vi "main.vi"() -> ()   [LabVIEW 2021]
uses:
  <extravilib>/ChannelInstances/Stream-c(dbl,dbl)/Read With Abort.vi
  <extravilib>/ChannelInstances/Stream-c(dbl,dbl)/Write With Abort.vi
  <extravilib>/ChannelInstances/Stream-c(dbl,dbl)/EndpointRead.vi
  <extravilib>/ChannelInstances/Stream-c(dbl,dbl)/Endpoint.vi
  <vilib>/Instr/_visa.llb/VISA Configure Serial Port (Instr).vi
  <extravilib>/ChannelInstances/Event Messenger-c(str)/Instantiate.vi
  <extravilib>/ChannelInstances/Event Messenger-c(str)/))Channel.vi
  <extravilib>/ChannelInstances/Stream-c(dbl,dbl)/Instantiate.vi
  <extravilib>/ChannelInstances/Stream-c(dbl,dbl)/)Channel.vi
  <resource>/ChannelSupport/_ChannelSupport/WaitIfNeeded.vi
  <extravilib>/ChannelInstances/Stream-c(dbl,dbl).lvlib
  <extravilib>/ChannelInstances/Event Messenger-c(str).lvlib
panel:
  in  "Start":bool
  out "File Path":path
  out "Recording?":bool
  in  "Record?":bool
  out "XY Graph":cluster{"X":dbl, "Y":dbl}[](graph)
  out "Temp":dbl
  out "Time":dbl
  in  "VISA resource name":refnum<visa-resource-name>
  in  "Stop":bool
  # "Select the VISA resource name before starting the application, you can choose to record to a file at any time using the checkbox. Data acquisition begins after you press Start."
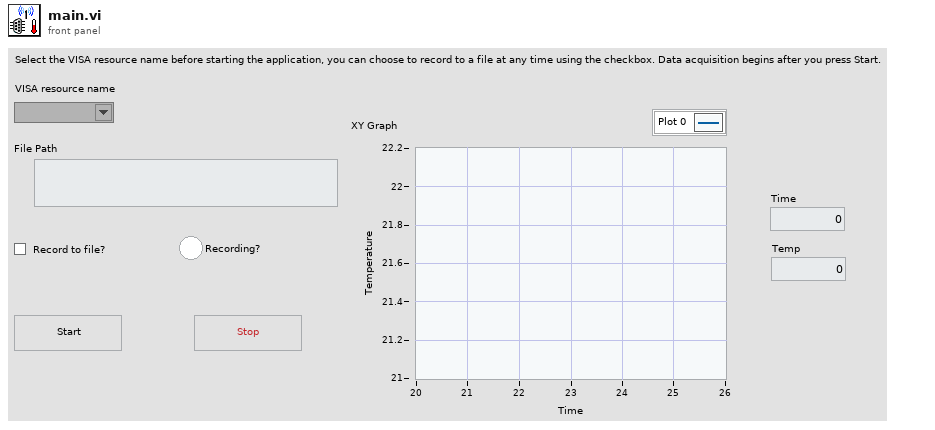
[diagram p1: front panel]
types:
  T1 = enum16{"open", "replace", "create", "open or create", "replace or create", "replace or create with confirmation"}
  T2 = typedef "Event Messenger-c(str).lvlib/))Channel.ctl" = refnum<queue>
  T3 = typedef "Stream-c(dbl,dbl).lvlib/)Channel.ctl" = refnum<queue>
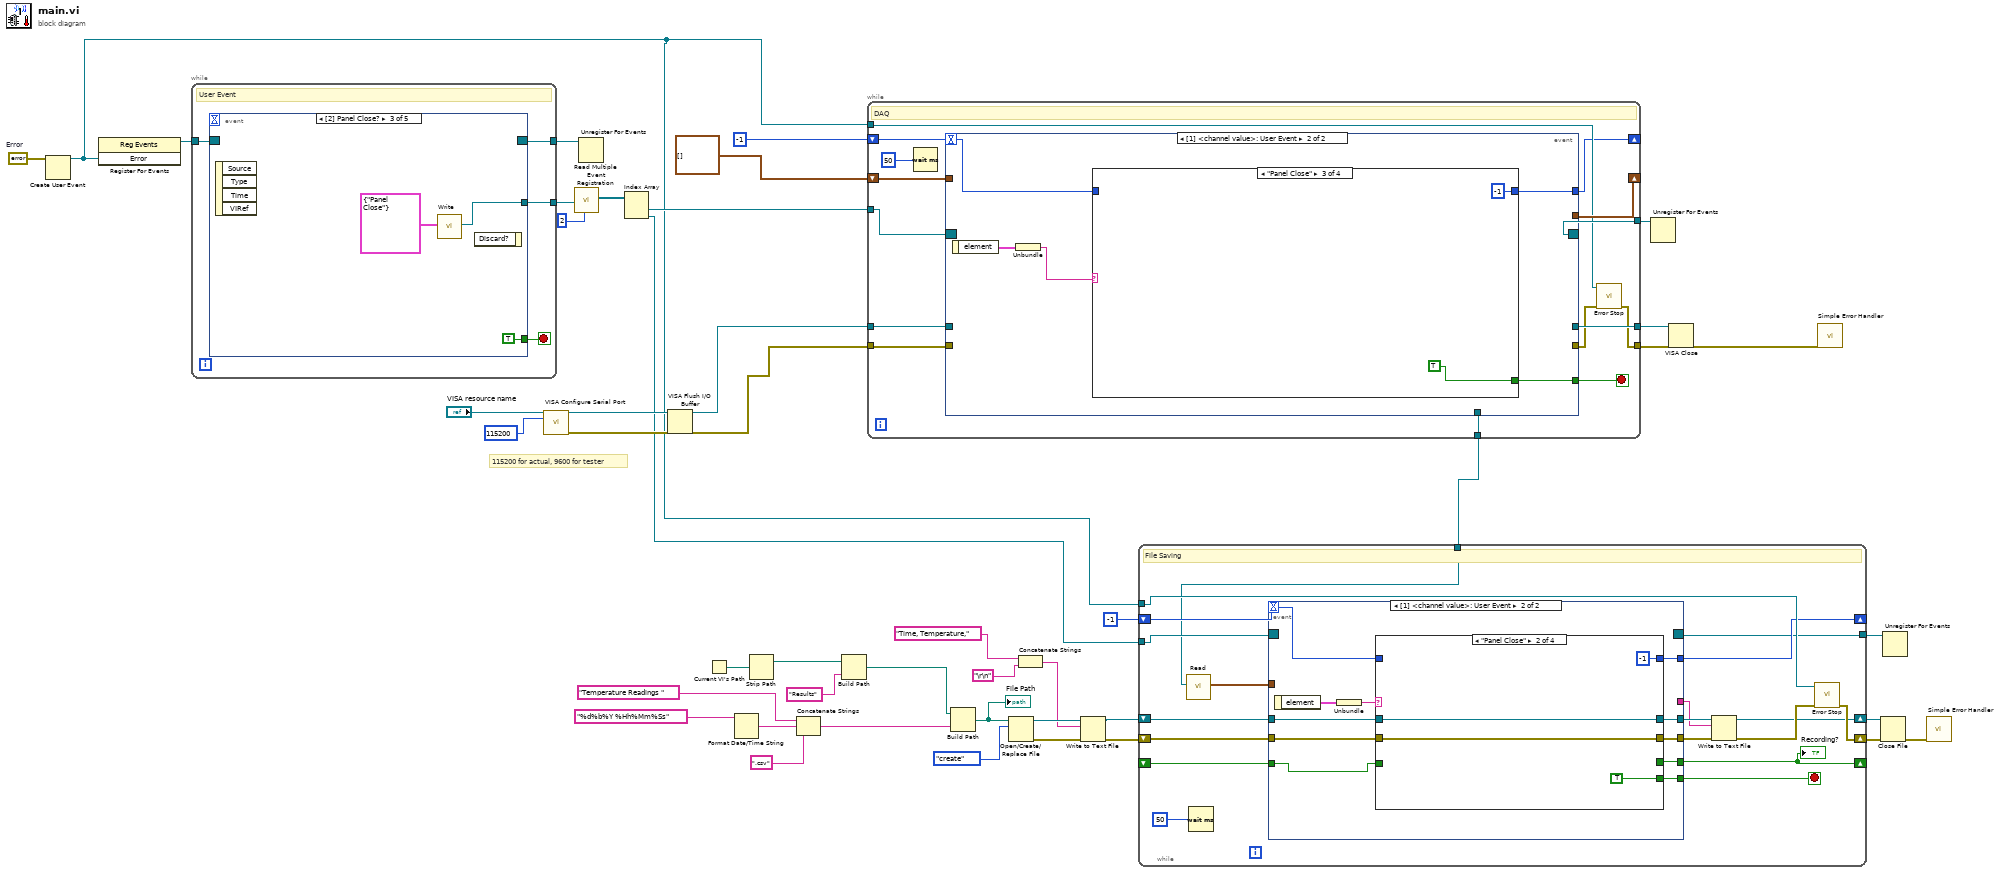
[diagram p0: block diagram]
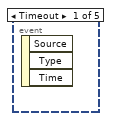
[diagram p2: hidden frame]
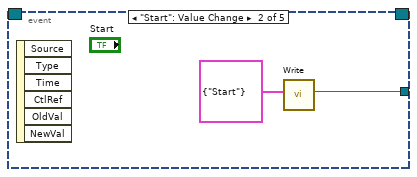
[diagram p3: hidden frame]
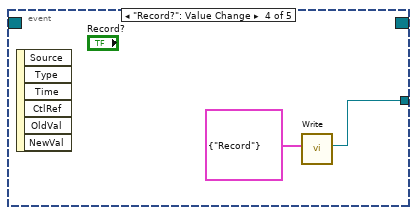
[diagram p4: hidden frame]
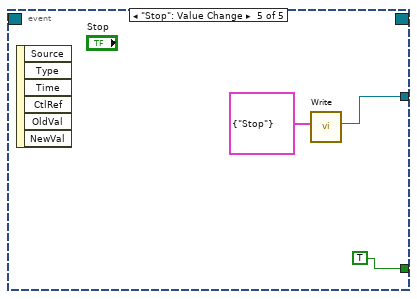
[diagram p5: hidden frame]
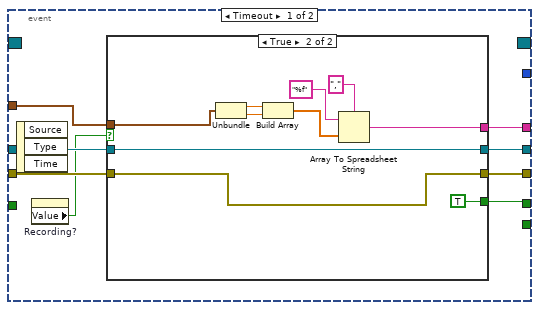
[diagram p6: hidden frame]
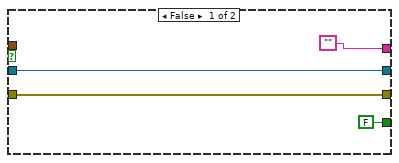
[diagram p7: hidden frame]
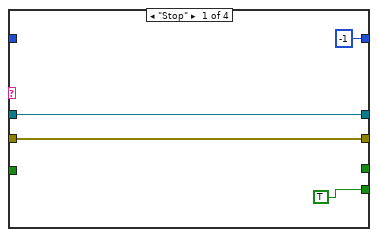
[diagram p8: hidden frame]
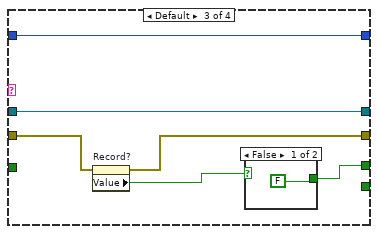
[diagram p9: hidden frame]
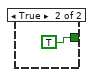
[diagram p10: hidden frame]
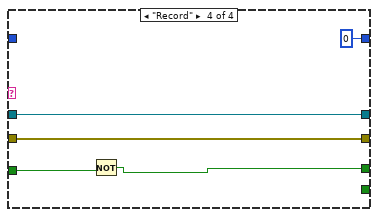
[diagram p11: hidden frame]
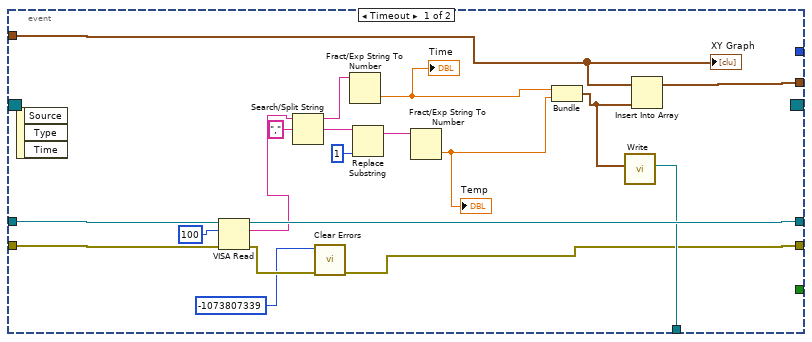
[diagram p12: hidden frame]
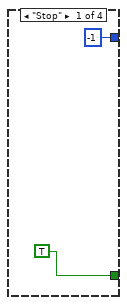
[diagram p13: hidden frame]
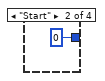
[diagram p14: hidden frame]
diagram:
  w5 = errorcluster {"status"=FALSE, "code"=0, "source"=""}  # Error
  # "115200 for actual, 9600 for tester"
  n1 = Create User Event(user event datatype=w5) -> (user event=w4:refnum<user-event>)  [unwired: 1 in, 1 out]
  n2 = register-events(w4) -> (reference out=w15:refnum<event-registration>)  [unwired: 2 in, 1 out]
  n3 = while {
    tunnel: w15 -> [w49]
    tunnel: [w48] -> w14
    tunnel: [w47] -> w13
    stop <- w46 stop-if-true
    # "User Event"
    n4 = event shown="[2] Panel Close?" {
      selector: w49 -> [_ _ _ _ _]
      dyn-events: [_ _ _ _ _] -> w48
      timeout: _ -> [_ _ _ _ _]
      tunnel: [_ w50 w53 w55 w58] -> w47
      tunnel: [_ _ TRUE _ TRUE] -> w46
      event Timeout {
        n5 = event-data() -> ()  [unwired: 1 in, 3 out]
      }
      event "Start": Value Change {
        n6 = event-data() -> ()  [unwired: 1 in, 6 out]
        n7 = call <extravilib>:"Write.vi"("element"=cluster{string} {"Start"}) -> ("channel"=w50:T2)  [unwired: 9 in, 1 out]
      }
      event Panel Close? {
        n8 = event-data() -> ()  [unwired: 1 in, 4 out]
        n9 = call <extravilib>:"Write.vi"("element"=cluster{string} {"Panel Close"}) -> ("channel"=w53:T2)  [unwired: 9 in, 1 out]
        n10 = event-data() -> ()  [unwired: 2 in, 1 out]
      }
      event "Record?": Value Change {
        n11 = event-data() -> ()  [unwired: 1 in, 6 out]
        n12 = call <extravilib>:"Write.vi"("element"=cluster{string} {"Record"}) -> ("channel"=w55:T2)  [unwired: 9 in, 1 out]
      }
      event "Stop": Value Change {
        n13 = event-data() -> ()  [unwired: 1 in, 6 out]
        n14 = call <extravilib>:"Write.vi"("element"=cluster{string} {"Stop"}) -> ("channel"=w58:T2)  [unwired: 9 in, 1 out]
      }
    }
  }
  n15 = call-poly "VISA Configure Serial Port"("VISA resource name"="VISA resource name", "baud rate (9600)"=u32 115200) -> ("VISA resource name out"=w45:refnum<visa-resource-name>, "error out"=w44:errorcluster)  [unwired: 12 in]
  n16 = call <extravilib>:"Read Multiple Event Registration.vi"("number of event structures"=u16 2, "channel"=w13) -> ("event registration refnums"=w11:refnum<event-registration>[])  [unwired: 9 in]
  n17 = Unregister For Events(event registration refnum=w14) -> ()  [unwired: 1 in, 1 out]
  n18 = Index Array(array=w11) -> (element #1=w8:refnum<event-registration>, element #2=w6:refnum<event-registration>)  [unwired: 2 in]
  n19 = VISA Flush I/O Buffer(VISA resource name=w45, error in (no error)=w44) -> (VISA resource name out=w10:refnum<visa-resource-name>, error out=w9:errorcluster)  [unwired: 1 in]
  n20 = Current VI's Path() -> (path=w33:path)
  n21 = Format Date/Time String(time format string (%c)="%d%b%Y %Hh%Mm%Ss") -> (date/time string=w37:string)  [unwired: 2 in]
  n22 = Strip Path(path=w33) -> (stripped path=w16:path)  [unwired: 1 out]
  n23 = Concatenate Strings("Temperature Readings " ("string"), w37, ".csv" ("string")) -> (w35:string)
  n24 = Build Path(base path=w16, name or relative path="Results") -> (appended path=w34:path)
  n25 = while {
    tunnel: w9 -> [w74]
    tunnel: w10 -> [w73]
    tunnel: [w63] -> w42
    tunnel: [w72] -> w41
    shift-right: [w71] -> _
    shift-left: cluster{dbl, dbl}[] [] -> [w70]
    tunnel: [w69] -> w20
    tunnel: w8 -> [w68]
    tunnel: [w67] -> w7
    tunnel: w4 -> [w65]
    shift-right: [w61] -> _
    shift-left: -1 -> [w62]
    stop <- w66 stop-if-true
    # "DAQ"
    n26 = Wait (ms)(milliseconds to wait=u32 50) -> ()  [unwired: 1 out]
    n27 = event shown="[1] <channel value>: User Event" {
      selector: w68 -> [_ _]
      dyn-events: [_ _] -> w67
      timeout: w62 -> [_ w95]
      tunnel: w74 -> [w93 _]
      tunnel: w73 -> [w92 _]
      tunnel: [w91 _] -> w72
      tunnel: [w90 _] -> w71
      tunnel: w70 -> [w89 _]
      tunnel: [w88 _] -> w69
      tunnel: [w87 _] -> w64
      tunnel: [_ w96] -> w66
      tunnel: [_ w94] -> w61
      event Timeout {
        n28 = event-data() -> ()  [unwired: 1 in, 3 out]
        n29 = VISA Read(VISA resource name=w92, byte count=u32 100, error in (no error)=w93) -> (VISA resource name out=w91:refnum<visa-resource-name>, read buffer=w82:string, error out=w85:errorcluster)  [unwired: 1 out]
        n30 = Search/Split String(string=w82, search string/char (-)=",") -> (substring before match=w81:string, match + rest of string=w80:string)  [unwired: 1 in, 1 out]
        n31 = call <vilib>:"Clear Errors.vi"("error in (no error)"=w85, "specific error code to clear (0: all)"=-1073807339) -> ("error out"=w87:errorcluster)  [unwired: 4 in, 1 out]
        n32 = Fract/Exp String To Number(string=w81) -> (number=w77:dbl)  [unwired: 3 in, 1 out]
        "Time" <- w77
        n33 = Replace Substring(2:1 ("length (len. of substring)"), 5:w80) -> (1:w78:string)  [unwired: 2 in, 1 out]
        n34 = Fract/Exp String To Number(string=w78) -> (number=w76:dbl)  [unwired: 3 in, 1 out]
        "Temp" <- w76
        n35 = Bundle(w77, w76) -> (w75:cluster{dbl, dbl})  [unwired: 1 in]
        n36 = call <extravilib>:"Write.vi"("element"=w75) -> ("channel"=w88:T3)  [unwired: 8 in, 2 out]
        n37 = Insert Into Array(array=w89, new element=w75) -> (w90:cluster{dbl, dbl}[])  [unwired: 1 in]
        "XY Graph" <- w89
      }
      event User Event {
        n38 = event-data() -> ("element"=w98:cluster{string})  [unwired: 1 in]
        n39 = Unbundle(w98) -> (w97:string)
        n40 = case shown="\"Panel Close\"" w97 {
          tunnel: [TRUE _ TRUE _] -> w96
          tunnel: w95 -> [_ _ _ w104]
          tunnel: [-1 0 -1 w104] -> w94
          frame "Stop" {
          }
          frame "Start" {
          }
          frame "Panel Close" {
          }
          frame Default {
          }
        }
      }
    }
    n41 = call "Error Stop.vi"("error in"=w64, "user event"=w65) -> ("error out"=w63:errorcluster)  [unwired: 9 in]
  }
  n42 = Build Path(base path=w34, name or relative path=w35) -> (appended path=w17:path)
  "File Path" <- w17
  n43 = Open/Create/Replace File(file path (use dialog)=w17, operation (0:open)=T1."create") -> (refnum out=w31:refnum<file>, error out=w30:errorcluster)  [unwired: 4 in, 1 out]
  n44 = Concatenate Strings("Time, Temperature,", "\r\n") -> (w27:string)
  n45 = Write to Text File(file (use dialog)=w31, text=w27, error in=w30) -> (refnum out=w18:refnum<file>, error out=w25:errorcluster)  [unwired: 1 in, 1 out]
  n46 = while {
    shift-right: [w106] -> w22
    shift-left: w18 -> [w123]
    shift-right: [w119] -> w24
    shift-left: w25 -> [w122]
    tunnel: w20 -> [w112]
    tunnel: w6 -> [w121]
    tunnel: w4 -> [w120]
    shift-right: [w117] -> _
    shift-left: -1 -> [w118]
    shift-right: [w115] -> _
    shift-left: _ -> [w114]
    tunnel: [w105] -> w1
    stop <- w116 stop-if-true
    # "File Saving"
    n47 = call <extravilib>:"Read.vi"("channel"=w112) -> ("element"=w113:cluster{dbl, dbl})  [unwired: 6 in, 4 out]
    n48 = Wait (ms)(milliseconds to wait=u32 50) -> ()  [unwired: 1 out]
    n49 = event shown="[1] <channel value>: User Event" {
      selector: w121 -> [_ _]
      dyn-events: [_ _] -> w105
      timeout: w118 -> [_ w154]
      tunnel: w123 -> [w131 w147]
      tunnel: w122 -> [w130 w149]
      tunnel: [w125 w148] -> w110
      tunnel: [_ w153] -> w117
      tunnel: [_ w152] -> w116
      tunnel: [w129 w151] -> w115
      tunnel: w114 -> [_ w150]
      tunnel: w113 -> [w127 _]
      tunnel: [w126 w146] -> w108
      tunnel: [w124 _] -> w107
      event Timeout {
        n50 = event-data() -> ()  [unwired: 1 in, 3 out]
        n51 = property on="Recording?" class="Bool (strict)"() -> ("Value"=w128:bool)  [unwired: 2 in, 2 out]
        n52 = case shown="True" w128 {
          tunnel: w131 -> [w133 w138]
          tunnel: [w133 w138] -> w126
          tunnel: [w134 w137] -> w125
          tunnel: w130 -> [w134 w137]
          tunnel: [FALSE TRUE] -> w129
          tunnel: w127 -> [_ w139]
          tunnel: ["" w136] -> w124
          frame False {
          }
          frame True {
            n53 = Unbundle(w139) -> (w145:dbl, w144:dbl)
            n54 = Build Array(w145, w144) -> (w141:dbl[])
            n55 = Array To Spreadsheet String(delimiter (Tab)=",", array=w141, 3:"%f" ("format string")) -> (spreadsheet string=w136:string)
          }
        }
      }
      event User Event {
        n56 = event-data() -> ("element"=w156:cluster{string})  [unwired: 1 in]
        n57 = Unbundle(w156) -> (w155:string)
        n58 = case shown="\"Panel Close\"" w155 {
          tunnel: w154 -> [_ _ w170 _]
          tunnel: [-1 -1 w170 0] -> w153
          tunnel: [TRUE TRUE _ _] -> w152
          tunnel: [_ _ w165 w175] -> w151
          tunnel: w150 -> [_ _ _ w176]
          tunnel: w149 -> [w158 w161 w168 w174]
          tunnel: [w158 w161 w167 w174] -> w148
          tunnel: w147 -> [w157 w162 w169 w173]
          tunnel: [w157 w162 w169 w173] -> w146
          frame "Stop" {
          }
          frame "Panel Close" {
          }
          frame Default {
            n59 = property on="Record?" class="Bool (strict)"(error in=w168) -> (error out=w167:errorcluster, "Value"=w166:bool)  [unwired: 1 in, 1 out]
            n60 = case shown="False" w166 {
              tunnel: [FALSE TRUE] -> w165
              frame False {
              }
              frame True {
              }
            }
          }
          frame "Record" {
            n61 = Not(x=w176) -> (.not. x?=w175:bool)
          }
        }
      }
    }
    "Recording?" <- w115
    n62 = Write to Text File(file (use dialog)=w108, text=w107, error in=w110) -> (refnum out=w106:refnum<file>, error out=w109:errorcluster)  [unwired: 1 in, 1 out]
    n63 = call "Error Stop.vi"("error in"=w109, "user event"=w120) -> ("error out"=w119:errorcluster)  [unwired: 9 in]
  }
  n64 = Unregister For Events(event registration refnum=w7) -> ()  [unwired: 1 in, 1 out]
  n65 = VISA Close(VISA resource name=w41, error in (no error)=w42) -> (error out=w40:errorcluster)
  n66 = call <vilib>:"Simple Error Handler.vi"("error in (no error)"=w40) -> ()  [unwired: 4 in, 5 out]
  n67 = Close File(refnum=w22, error in=w24) -> (error out=w23:errorcluster)  [unwired: 1 out]
  n68 = Unregister For Events(event registration refnum=w1) -> ()  [unwired: 1 in, 1 out]
  n69 = call <vilib>:"Simple Error Handler.vi"("error in (no error)"=w23) -> ()  [unwired: 4 in, 5 out]
